vi "Supply_SetVolts.vi"(8 "error in (no error)":errorcluster, 9 "Command string":string, 10 "Volts IN [V]":dbl, 11 "KE237 in":refnum<class "KE237.lvclass">) -> (0 "error out":errorcluster, 2 "Compliance exceeded?":bool, 3 "KE237. out":refnum<class "KE237.lvclass">)   [LabVIEW 2018, in "KE237.lvclass"]
uses:
  KE237.lvclass
  SupplyControl.lvclass
panel:
  out "Command sent":string
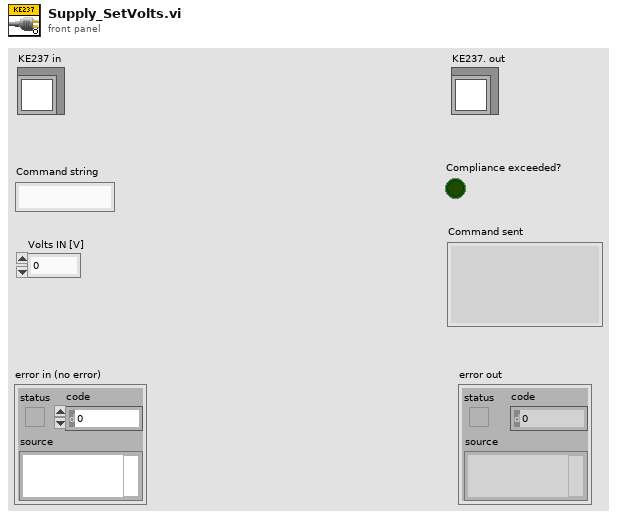
[diagram p1: front panel]
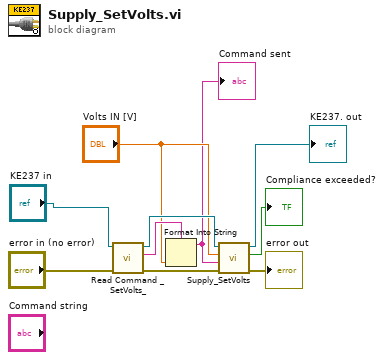
[diagram p0: block diagram]
diagram:
  n1 = call-dynamic "Read Command _SetVolts_.vi"("error in (no error)"="error in (no error)", "SupplyControl in"="KE237 in") -> ("error out"=w6:errorcluster, "Command \"SetVolts\""=w7:string, "SupplyControl out"=w5:refnum<class "KE237.lvclass">)  [unwired: 7 in]
  n2 = Format Into String(format string=w7, "Volts IN [V]") -> (resulting string=w3:string)  [unwired: 2 in, 1 out]
  "Command sent" <- w3
  n3 = call-parent "Supply_SetVolts.vi"("error in (no error)"=w6, "Command string"=w3, "Volts IN [V]"="Volts IN [V]", "SupplyControl in"=w5) -> ("error out"=→"error out":errorcluster, "Compliance exceeded?"=→"Compliance exceeded?":bool, "SupplyControl out"=→"KE237. out":refnum<class "KE237.lvclass">)  [unwired: 5 in]
